vi "Expand Universe.vi"(0 "Universe":string[][](array[string]), 1 "Space (.)":string=".", 2 "Expansion Rate (2x)":i32=2) -> (3 "Expanded Universe":string[][](array[string]))   [LabVIEW 2020, in "AoC 2023.lvlib"]
uses:
  AoC 2023.lvlib
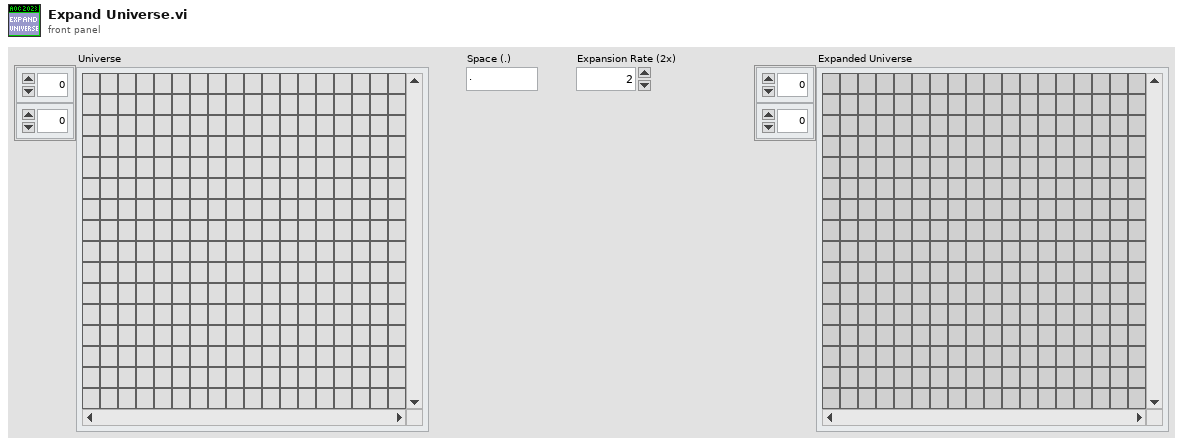
[diagram p1: front panel]
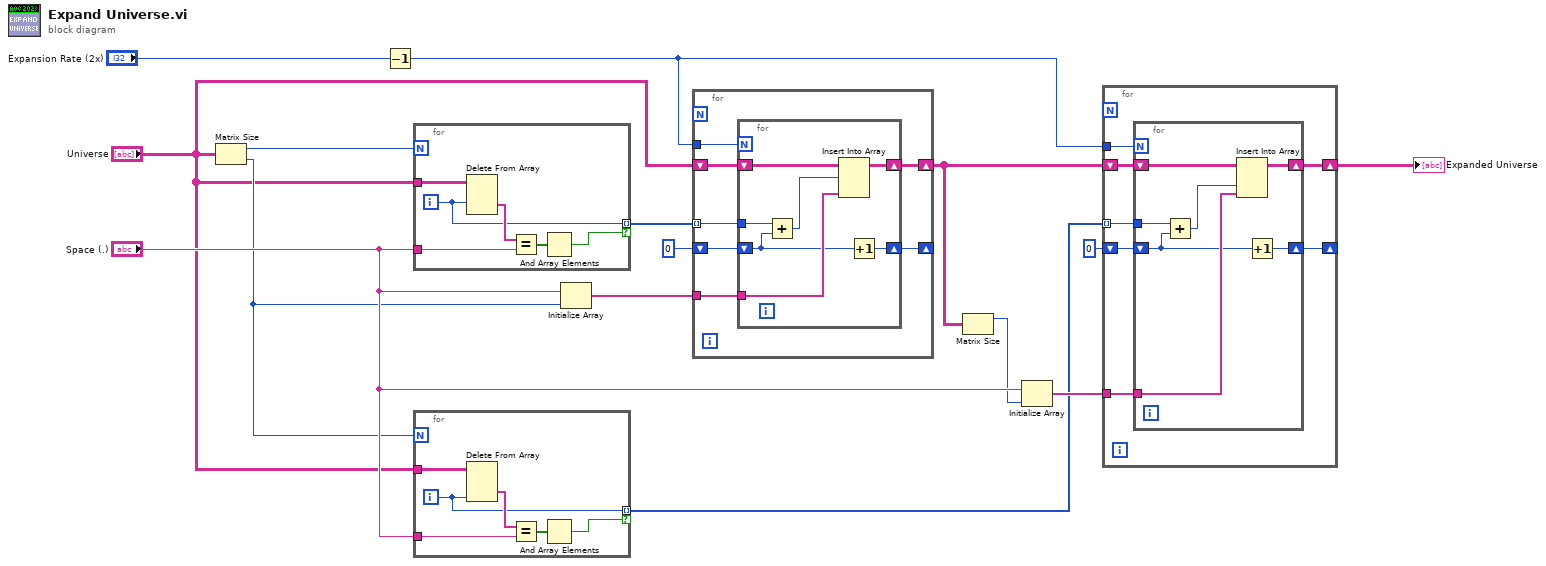
[diagram p0: block diagram]
diagram:
  n1 = Matrix Size(0:"Universe") -> (1:w3:i32, 2:w8:i32)
  n2 = Decrement(x="Expansion Rate (2x)") -> (x-1=w1:i32)
  n3 = for {
    N: w3 -> [_]
    tunnel: "Universe" -> [w21]
    tunnel: [w19] -> w4 mode=indexing if=w16
    tunnel: "Space (.)" -> [w18]
    i -> [w19]
    n4 = Delete From Array(array=w21, index (row)=w19) -> (deleted portion=w20:string[])  [unwired: 2 in, 1 out]
    n5 = Equal?(x=w20, y=w18) -> (x = y?=w17:bool[])
    n6 = And Array Elements(Boolean array=w17) -> (logical AND=w16:bool)
  }
  n7 = for {
    N: w8 -> [_]
    tunnel: "Universe" -> [w27]
    tunnel: [w22] -> w10 mode=indexing if=w23
    tunnel: "Space (.)" -> [w25]
    i -> [w22]
    n8 = Delete From Array(array=w27, index (col)=w22) -> (deleted portion=w26:string[])  [unwired: 2 in, 1 out]
    n9 = Equal?(x=w26, y=w25) -> (x = y?=w24:bool[])
    n10 = And Array Elements(Boolean array=w24) -> (logical AND=w23:bool)
  }
  n11 = Initialize Array("Space (.)", w8) -> (w9:string[])
  n12 = for {
    shift-right: [w32] -> w11
    shift-left: "Universe" -> [w33]
    tunnel: w4 -> [w30] mode=indexing
    tunnel: w9 -> [w31]
    shift-right: [w34] -> _
    shift-left: 0 -> [w29]
    tunnel: w1 -> [w28]
    n13 = for {
      N: w28 -> [_]
      tunnel: w31 -> [w38]
      tunnel: w30 -> [w37]
      shift-right: [w41] -> w34
      shift-left: w29 -> [w36]
      shift-right: [w39] -> w32
      shift-left: w33 -> [w40]
      n14 = Add(x=w37, y=w36) -> (x+y=w35:i32)
      n15 = Insert Into Array(array=w40, index (row)=w35, new element=w38) -> (w39:string[][])  [unwired: 1 in]
      n16 = Increment(x=w36) -> (x+1=w41:i32)
    }
  }
  n17 = Matrix Size(0:w11) -> (1:w12:i32)  [unwired: 1 out]
  n18 = Initialize Array("Space (.)", w12) -> (w14:string[])
  n19 = for {
    shift-right: [w46] -> w15
    shift-left: w11 -> [w47]
    tunnel: w10 -> [w44] mode=indexing
    tunnel: w14 -> [w45]
    shift-right: [w48] -> _
    shift-left: 0 -> [w43]
    tunnel: w1 -> [w42]
    n20 = for {
      N: w42 -> [_]
      tunnel: w45 -> [w52]
      tunnel: w44 -> [w51]
      shift-right: [w55] -> w48
      shift-left: w43 -> [w50]
      shift-right: [w53] -> w46
      shift-left: w47 -> [w54]
      n21 = Add(x=w51, y=w50) -> (x+y=w49:i32)
      n22 = Insert Into Array(array=w54, index (col)=w49, new element=w52) -> (w53:string[][])  [unwired: 1 in]
      n23 = Increment(x=w50) -> (x+1=w55:i32)
    }
  }
  "Expanded Universe" <- w15
